vi "OAT Polar Plot.vi"   [LabVIEW 2017]
doc: "Draws a polar plot on a picture control and adds labels. The polar plot displays the magnitude and phase of a certain order on a picture control. You must manually select the polymorphic instance to use. Use the Manual Label instance if you want to label the polar plot manually."
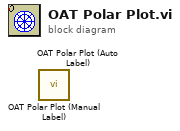
[diagram p0: block diagram]
diagram:
  n1 = call <vilib>:"OAT Polar Plot (Manual Label).vi"() -> ()  [unwired: 13 in, 3 out]
  n2 = call <vilib>:"OAT Polar Plot (Auto Label).vi"() -> ()  [unwired: 14 in, 2 out]
